vi "init.vi"(8 "error in (no error)":errorcluster, 10 "baudRate":u32, 11 "deviceName":string) -> (0 "error out":errorcluster, 2 "return type":i32, 3 "pHandle":u32)   [LabVIEW 2011, in "sbgLabView.lvlib"]
uses:
  sbgLabView.lvlib
  sbgMatLab.dll
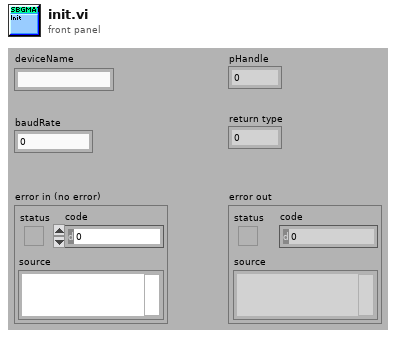
[diagram p1: front panel]
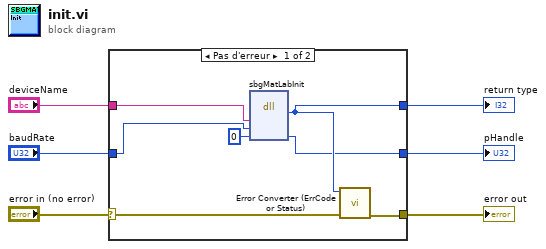
[diagram p0: block diagram]
diagram:
  n1 = case shown="Pas d'erreur" "error in (no error)" {
    selector: "error in (no error)" -> [w8 w14]
    tunnel: [w7 w14] -> w5
    tunnel: [w13 _] -> w4
    tunnel: "deviceName" -> [w12 _]
    tunnel: "baudRate" -> [w11 _]
    tunnel: [w9 _] -> w1
    frame No Error {
      n2 = dll-call lib="C:/SBG-Systems/remote/projects/software/projects/labviewExample/sbgLabView/sbgMatLab.*" fn="sbgMatLabInit"("deviceName"=w12, "baudRate"=w11, "pHandle"=u32 0) -> (w13:i32, "pHandle"=w9:u32)  [unwired: 5 in, 2 out]
      n3 = call "Error Converter (ErrCode or Status).vi"("error in (no error)"=w8, "error code"=w13) -> ("error out"=w7:errorcluster)  [unwired: 9 in]
    }
    frame Error {
    }
  }
  "return type" <- w4
  "pHandle" <- w1
  "error out" <- w5
